vi "模块启用配置框.vi"() -> ()   [LabVIEW 2016]
uses:
  <vilib>/Utility/config.llb/NI_LVConfig.lvlib
panel:
  in  "取消":bool
  in  "确认":bool
  in  "CODMn启用":bool caption="CODMn禁用"
  in  "质控单元启用":bool caption="质控单元禁用"
  in  "总磷总氮启用":bool caption="总磷总氮禁用"
  in  "流量计启用":bool caption="流量计禁用"
  in  "氨氮启用":bool caption="氨氮禁用"
  in  "多参数启用":bool caption="多参数禁用"
  in  "CODcr启用":bool caption="CODcr禁用"
  # "模块启用配置"
  # "说明:\n选择所需要启动的模块,并按确认,软件将重启生效."
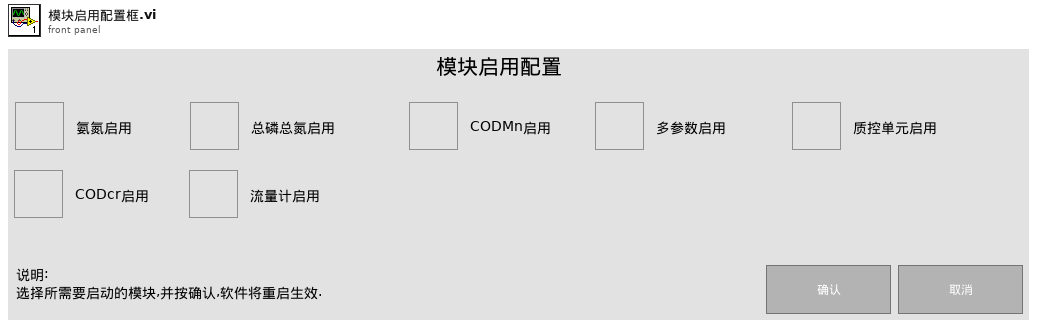
[diagram p1: front panel]
types:
  T1 = typedef "NI_LVConfig.lvlib/Config Data RefNum.ctl" = refnum<k1>
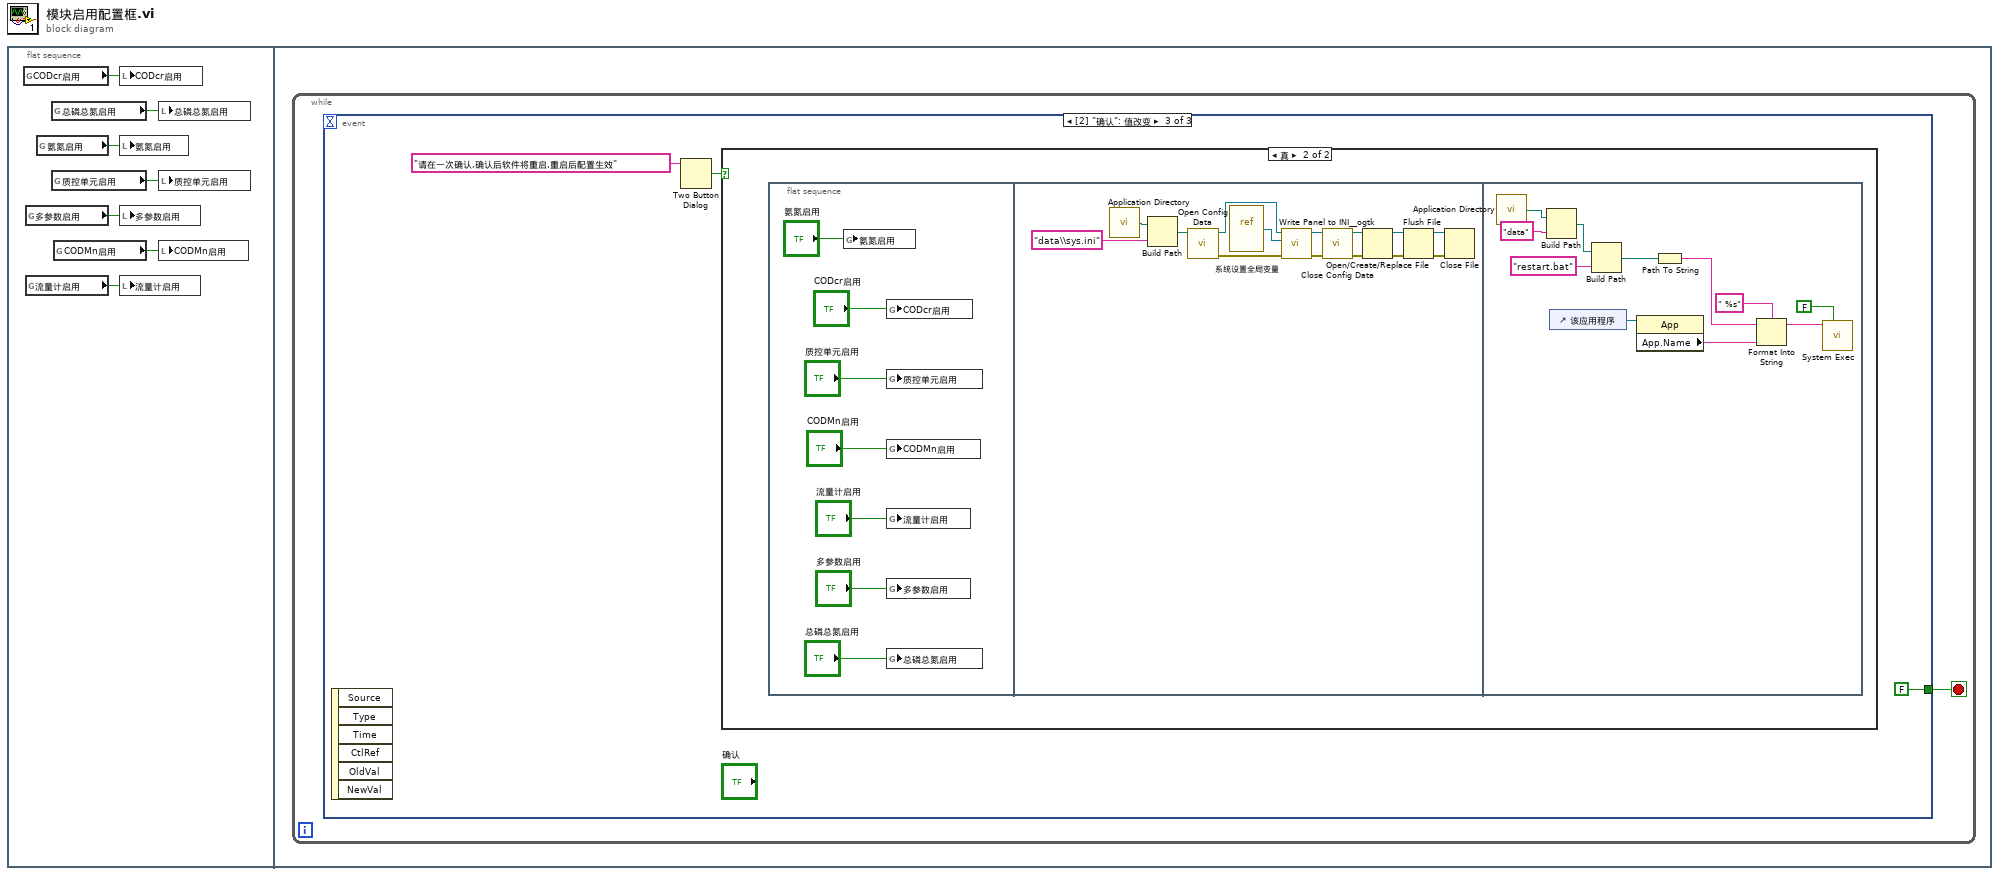
[diagram p0: block diagram]
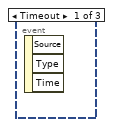
[diagram p2: hidden frame]
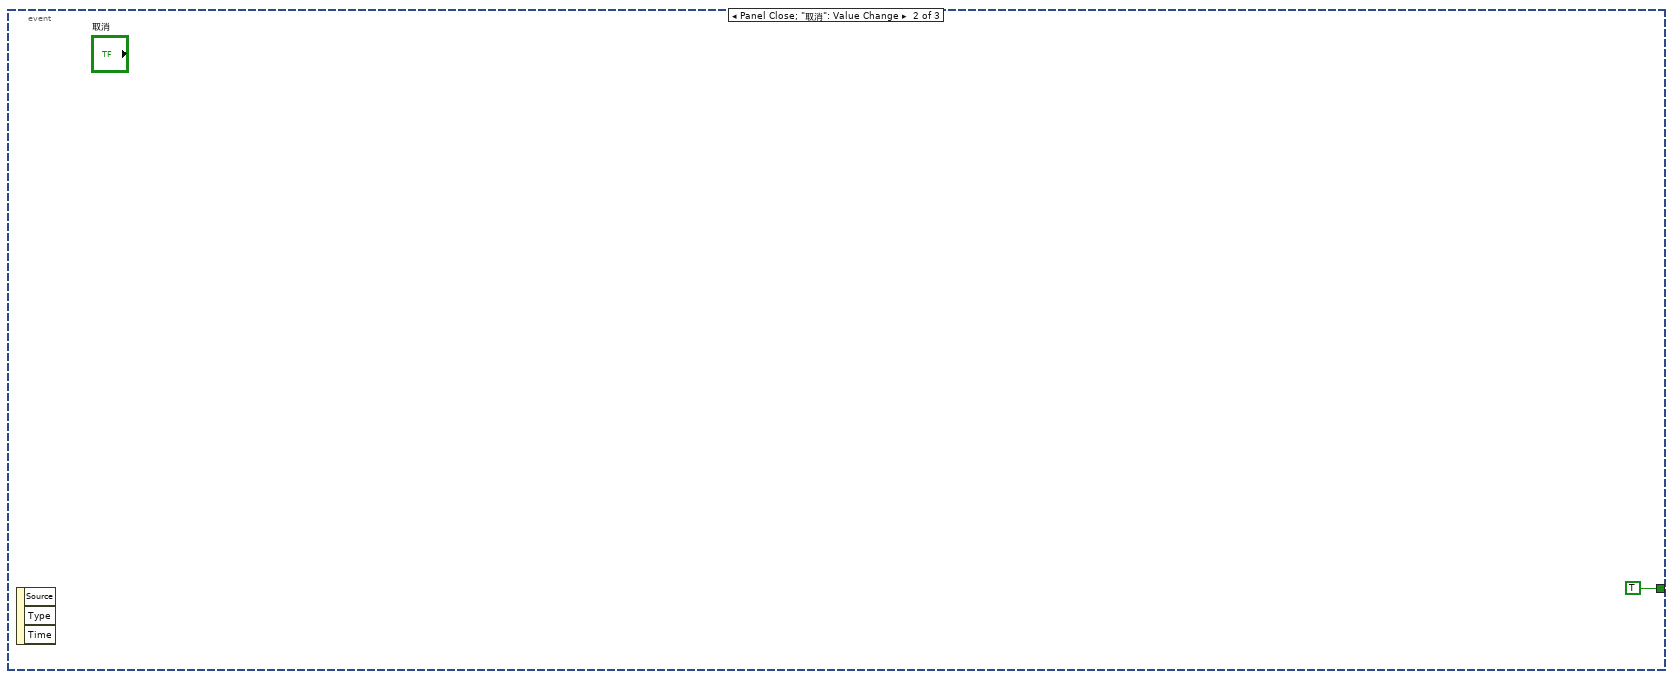
[diagram p3: hidden frame]
diagram:
  n1 = flat-sequence {
    frame #0 {
      n2 = global read "系统设置全局变量.vi" "CODcr启用"() -> (w7:bool)
      n3 = global read "系统设置全局变量.vi" "多参数启用"() -> (w5:bool)
      n4 = global read "系统设置全局变量.vi" "流量计启用"() -> (w4:bool)
      n5 = global read "系统设置全局变量.vi" "氨氮启用"() -> (w3:bool)
      n6 = global read "系统设置全局变量.vi" "总磷总氮启用"() -> (w6:bool)
      n7 = global read "系统设置全局变量.vi" "质控单元启用"() -> (w1:bool)
      n8 = global read "系统设置全局变量.vi" "CODMn启用"() -> (w2:bool)
      n9 = local write "CODcr启用"(w7) -> ()
      n10 = local write "氨氮启用"(w3) -> ()
      n11 = local write "多参数启用"(w5) -> ()
      n12 = local write "流量计启用"(w4) -> ()
      n13 = local write "总磷总氮启用"(w6) -> ()
      n14 = local write "质控单元启用"(w1) -> ()
      n15 = local write "CODMn启用"(w2) -> ()
    }
    frame #1 {
      n16 = while {
        stop <- w8 stop-if-true
        n17 = event shown="[2] \"确认\": 值改变" {
          selector: _ -> [_ _ _]
          dyn-events: _ -> [_ _ _]
          timeout: _ -> [_ _ _]
          tunnel: [_ TRUE FALSE] -> w8
          event Timeout {
            n18 = event-data() -> ()  [unwired: 1 in, 3 out]
          }
          event Panel Close; "取消": Value Change {
            n19 = event-data() -> ()  [unwired: 1 in, 3 out]
          }
          event "确认": Value Change {
            n20 = event-data() -> ()  [unwired: 1 in, 6 out]
            n21 = Two Button Dialog(message="请在一次确认,确认后软件将重启,重启后配置生效" ("消息")) -> (T button?=w10:bool)  [unwired: 2 in]
            n22 = case shown="真" w10 {
              frame False {
              }
              frame True {
                n23 = flat-sequence {
                  frame #0 {
                    n24 = global write "系统设置全局变量.vi" "氨氮启用"("氨氮启用") -> ()
                    n25 = global write "系统设置全局变量.vi" "CODcr启用"("CODcr启用") -> ()
                    n26 = global write "系统设置全局变量.vi" "质控单元启用"("质控单元启用") -> ()
                    n27 = global write "系统设置全局变量.vi" "CODMn启用"("CODMn启用") -> ()
                    n28 = global write "系统设置全局变量.vi" "流量计启用"("流量计启用") -> ()
                    n29 = global write "系统设置全局变量.vi" "多参数启用"("多参数启用") -> ()
                    n30 = global write "系统设置全局变量.vi" "总磷总氮启用"("总磷总氮启用") -> ()
                  }
                  frame #1 {
                    n31 = call <vilib>:"Application Directory.vi"() -> ("Application Directory"=w33:path)
                    n32 = Build Path(base path=w33, name or relative path="data\\sys.ini" ("名称或相对路径")) -> (appended path=w31:path)
                    n33 = call <vilib>:"Open Config Data.vi"("configuration file path"=w31) -> ("error out"=w27:errorcluster, "refnum"=w30:T1)  [unwired: 8 in, 1 out]
                    n34 = vi-ref "系统设置全局变量.vi"() -> (w29:refnum<vi>)
                    n35 = call <userlib>:"Write Panel to INI__ogtk.vi"("error in (no error)"=w27, "VI ref"=w29, "refnum"=w30) -> ("error out"=w26:errorcluster, "refnum out"=w28:T1)  [unwired: 7 in]
                    n36 = call <vilib>:"Close Config Data.vi"("error in (no error)"=w26, "refnum"=w28) -> ("error out"=w21:errorcluster, "file path"=w20:path)  [unwired: 8 in]
                    n37 = Open/Create/Replace File(file path (use dialog)=w20, error in=w21) -> (refnum out=w24:refnum<file>, error out=w25:errorcluster)  [unwired: 4 in, 1 out]
                    n38 = Flush File(refnum=w24, error in=w25) -> (refnum out=w23:refnum<file>, error out=w22:errorcluster)
                    n39 = Close File(refnum=w23, error in=w22) -> ()  [unwired: 2 out]
                  }
                  frame #2 {
                    n40 = call <vilib>:"Application Directory.vi"() -> ("Application Directory"=w43:path)
                    n41 = Build Path(base path=w43, name or relative path="data" ("名称或相对路径")) -> (appended path=w41:path)
                    n42 = control-ref of="该应用程序"() -> (w44:refnum<vi>)
                    n43 = Build Path(base path=w41, name or relative path="restart.bat" ("名称或相对路径")) -> (appended path=w39:path)
                    n44 = property class="App"(reference=w44) -> ("App.Name"=w36:string)  [unwired: 1 in, 2 out]
                    n45 = Path To String(path=w39) -> (string=w38:string)
                    n46 = Format Into String(format string=" %s" ("格式字符串"), initial string=w38, w36) -> (resulting string=w35:string)  [unwired: 1 in, 1 out]
                    n47 = call <vilib>:"System Exec.vi"("wait until completion? (T)"=FALSE, "command line"=w35) -> ()  [unwired: 6 in, 4 out]
                  }
                }
              }
            }
          }
        }
      }
    }
  }
